vi "Measurement Logic.vi"() -> ()   [LabVIEW 2024, in "Line Regulation_Channel Ganging.lvlib"]
uses:
  Line Regulation_Channel Ganging.lvlib
  <vilib>/Plug-In SDKs/Measurements/Measure Call Context/Measure Call Context.lvclass
  Measurement Configuration.ctl
  Measurement Results.ctl
  <instrlib>/niDCPower/nidcpower.llb/niDCPower Source Mode.ctl
  <instrlib>/niDCPower/nidcpower.llb/niDCPower Wait For Event - Event.ctl
  <instrlib>/niDCPower/nidcpower.llb/niDCPower Output Function.ctl
  shared subVIs/Triggers and Events/NIDCPower_channel_ganging - Configure Digital Edge Source Trigger.vi
  shared subVIs/Triggers and Events/NIDCPower_channel_ganging - Configure Digital Edge Measure Trigger.vi
panel:
  out "measurement results":T1
  in  "measurement configuration":T2={"Source master resource name"="", "Load master resource name"="", "Source slave resource names"=["", ""], "Load slave resource names"=["", ""], "Source system configuration"=enum."Parallel", "Source voltage level range"=64.0, "Source limit symmetry"=enum."Asymmetric", "Source current limit range"=-32.0, "Source current limit low"=-64.0, "Source current limit high"=-64.0, "Source transient response"=1038, "Source sense"=1008, "Source start voltage"=1.0, "Source current sweep points/points per decade"=1, "Source stop voltage"=14.0, "Source voltage gain bandwidth"=2000.0, "Source voltage compensation frequency"=3530.0, "Source voltage pole-zero ratio"=2.0, "Load system configuration"=enum."Parallel", "Load current level"=50.0, "Load current level range"=80.0, "Load limit symmetry"=enum."Symmetric", "Load voltage limit range"=6.0, "Load voltage limit low"=0.0, "Load voltage limit high"=inf, "Load transient response"=1038, "Load sense"=1009, "DUT setup time"=1.0, "Source delay"=0.005, "Aperture time"=0.005, "Load current gain bandwidth"=14000.0, "Load current compensation frequency"=180000.0, "Load current pole-zero ratio"=0.3, "Nominal output voltage"=0.005, "Source sweep type"="Logarithmic", "Mode of operation"=enum."Power on the DUT", "Measurement timeout"=0.0} {"Measurement timeout" format="%.3ps"; "Load sense" items=["Local"=1008, "Remote"=1009]; "Load transient response" items=["Slow"=1041, "Normal"=1038, "Fast"=1039, "Custom"=1042]; "Load voltage limit high" format="%#_6p"; "Load voltage limit low" format="%#_6p"; "Load voltage limit range" format="%#_6p"; "Load current level range" format="%#_6p"; "Source start voltage" format="%#_6p"; "Source sense" items=["Local"=1008, "Remote"=1009]; "Source transient response" items=["Slow"=1041, "Normal"=1038, "Fast"=1039, "Custom"=1042]; "Source current limit low" format="%#_6p"}
  out "measure call context out":refnum<class "Measure Call Context.lvclass">
  in  "measure call context in":refnum<class "Measure Call Context.lvclass">
  out "error out":errorcluster
  in  "error in":errorcluster
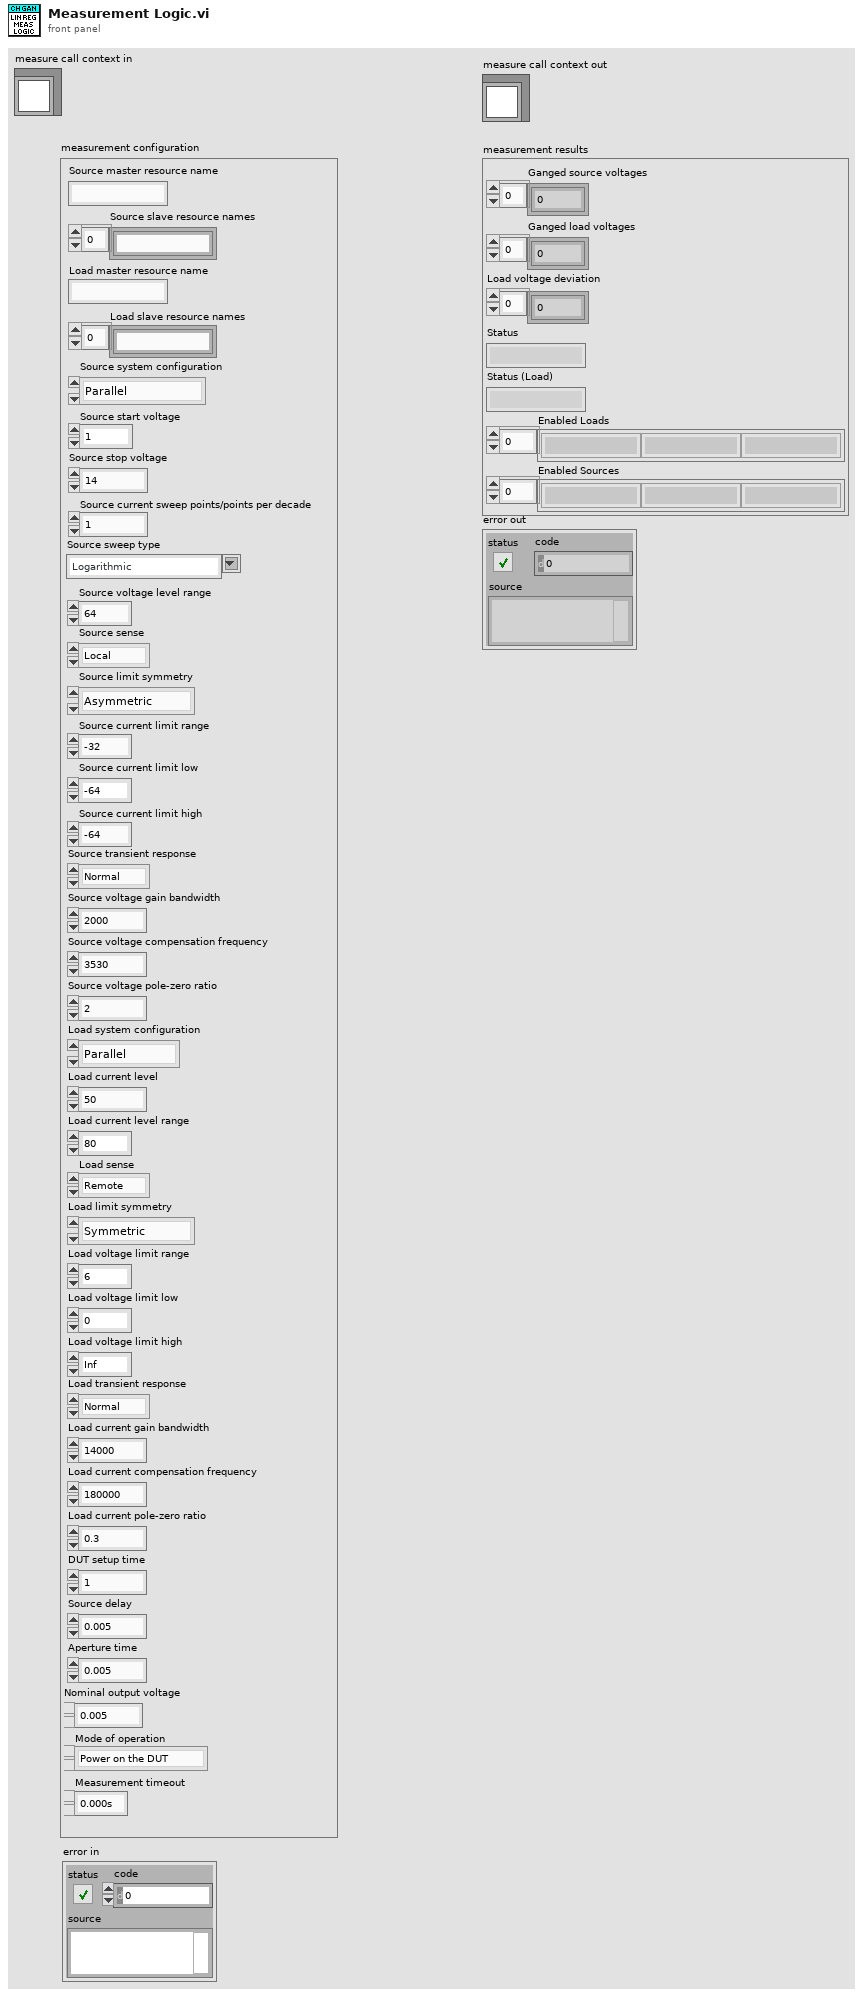
[diagram p1: front panel]
types:
  T1 = typedef "Line Regulation_Channel Ganging.lvlib/Measurement Results.ctl" = cluster{"Ganged source voltages":dbl[], "Ganged load voltages":dbl[], "Load voltage deviation":dbl[], "Status":string, "Status (Load)":string, "Enabled Loads":string[], "Enabled Sources":string[]}
  T2 = typedef "Line Regulation_Channel Ganging.lvlib/Measurement Configuration.ctl" = cluster{"Source master resource name":string, "Load master resource name":string, "Source slave resource names":string[], "Load slave resource names":string[], "Source system configuration":enum32{"Series", "Parallel", "Manual"}, "Source voltage level range":dbl, "Source limit symmetry":enum32{"Symmetric", "Asymmetric"}, "Source current limit range":dbl, "Source current limit low":dbl, "Source current limit high":dbl, "Source transient response":i32, "Source sense":i32, "Source start voltage":dbl, "Source current sweep points/points per decade":i32, "Source stop voltage":dbl, "Source voltage gain bandwidth":dbl, "Source voltage compensation frequency":dbl, "Source voltage pole-zero ratio":dbl, "Load system configuration":enum32{"Series", "Parallel", "Manual"}, "Load current level":dbl, "Load current level range":dbl, "Load limit symmetry":enum32{"Symmetric", "Asymmetric"}, "Load voltage limit range":dbl, "Load voltage limit low":dbl, "Load voltage limit high":dbl, "Load transient response":i32, "Load sense":i32, "DUT setup time":dbl, "Source delay":dbl, "Aperture time":dbl, "Load current gain bandwidth":dbl, "Load current compensation frequency":dbl, "Load current pole-zero ratio":dbl, "Nominal output voltage":dbl, "Source sweep type":string, "Mode of operation":enum32{"Power on the DUT", "Perform measurement", "Power off the DUT"}, "Measurement timeout":dbl}
  T3 = enum32{"Power on the DUT", "Perform measurement", "Power off the DUT"}
  T4 = typedef "niDCPower Output Function.ctl" = i32
  T5 = typedef "niDCPower Source Mode.ctl" = i32
  T6 = typedef "NIDCPower_channel_ganging - ctl - channel def.ctl" = cluster{"resource name":refnum<k15>, "channels":string, "Channel Mode":T7}
  T7 = typedef "NIDCPower_channel_ganging - ctl - channel mode.ctl" = enum32{"Master", "Slave", "Slave - Inverted"}
  T8 = typedef "NIDCPower_channel_ganging - ctl - ganged session.ctl" = cluster{"Ganged Config":T9, "Session List":refnum<k15>[], "Session Mode":T7[], "Channel":string[]}
  T9 = typedef "NIDCPower_channel_ganging - ctl - ganged config.ctl" = enum32{"Series", "Parallel", "Manual"}
  T10 = typedef "niDCPower Wait For Event - Event.ctl" = i32
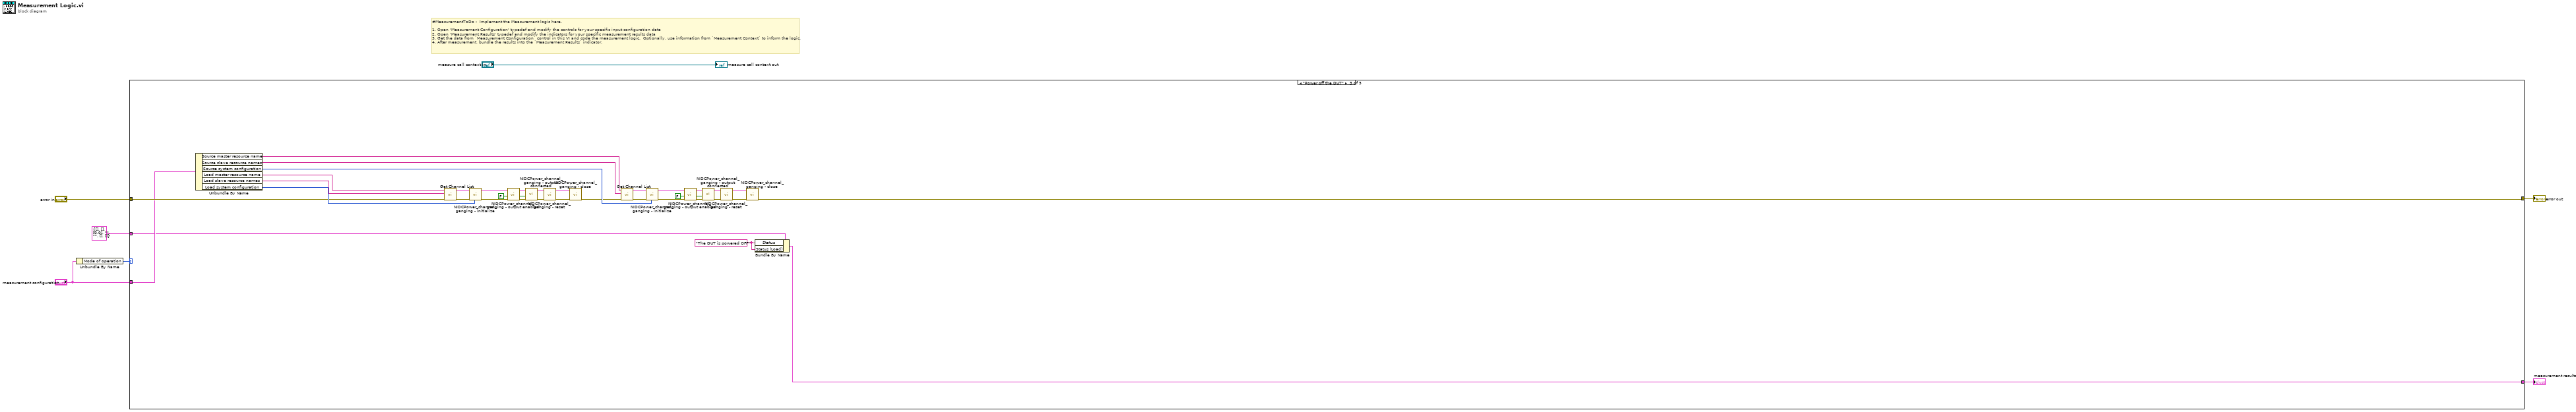
[diagram p0: block diagram]
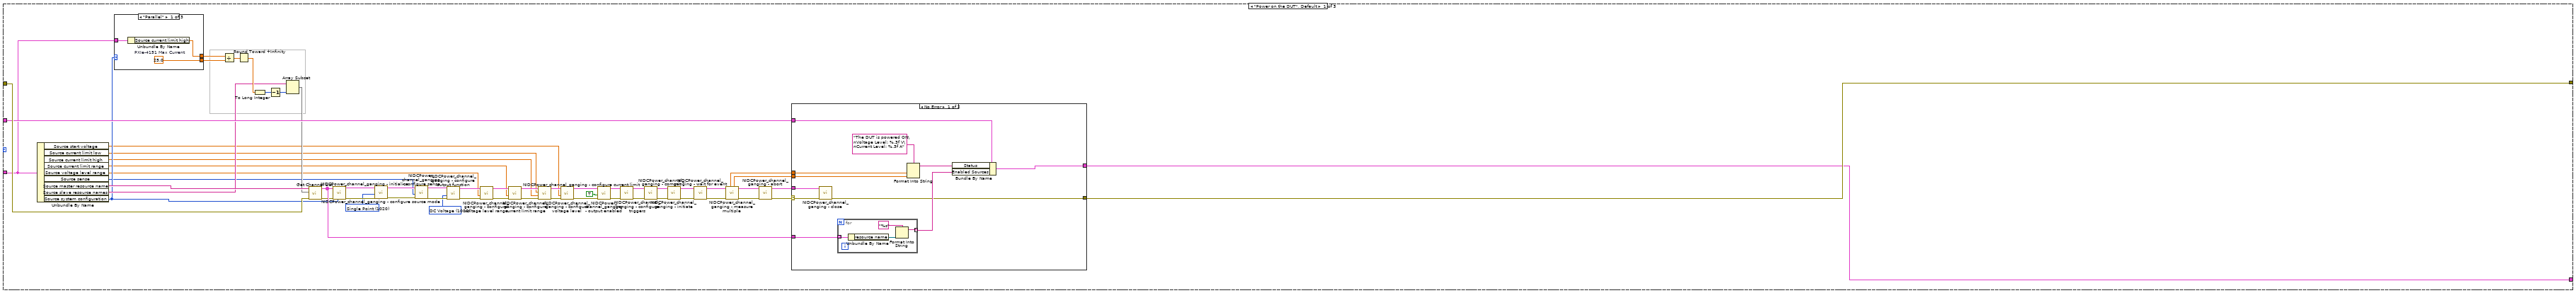
[diagram p2: hidden frame]
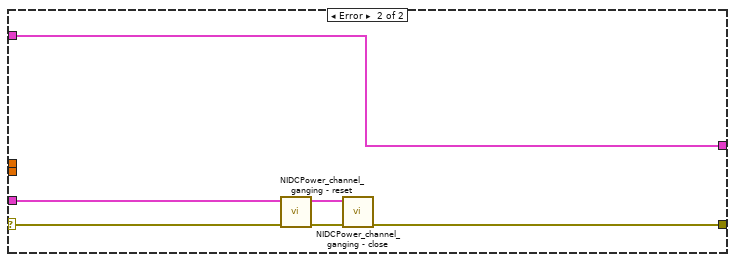
[diagram p3: hidden frame]
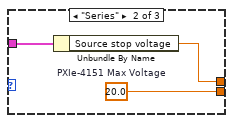
[diagram p4: hidden frame]
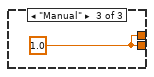
[diagram p5: hidden frame]
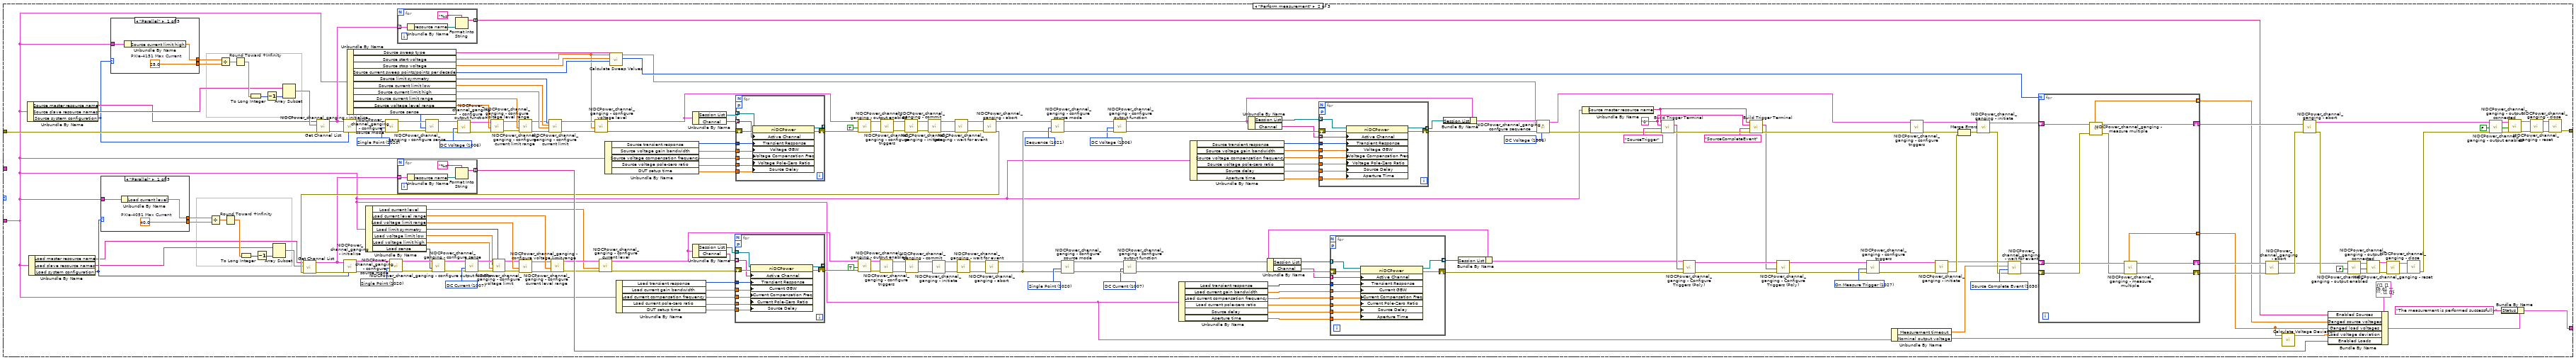
[diagram p6: hidden frame]
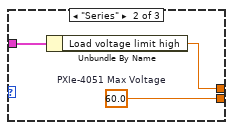
[diagram p7: hidden frame]
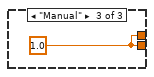
[diagram p8: hidden frame]
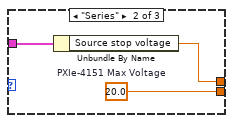
[diagram p9: hidden frame]
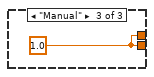
[diagram p10: hidden frame]
diagram:
  # "#MeasurementToDo :  Implement the Measurement logic here.\n\n1. Open 'Measurement Configuration' typedef and modify the controls for your specific input configuration data\n2. Open 'Measurement Results' typedef and modify the indicators for your specific measurement results data\n3. Get the data from `Measurement Configuration` control in this VI and code the measurement logic.  Optionally, use information from `Measurement Context` to inform the logic.\n4. After measurement, bundle the results into the `Measurement Results` indicator."
  n1 = Unbundle By Name("measurement configuration") -> ("Mode of operation"=w3:T3)
  n2 = case shown="\"Power off the DUT\"" w3 {
    tunnel: [w8 w94 w387] -> w6
    tunnel: "measurement configuration" -> [w53 w99 w389]
    tunnel: [w9 w121 w386] -> w5
    tunnel: "error in" -> [w65 w120 w390]
    tunnel: T1 {"Ganged source voltages"=[], "Ganged load voltages"=[], "Load voltage deviation"=[0.0], "Status"="", "Status (Load)"="", "Enabled Loads"=[], "Enabled Sources"=[]} ("Measurement Results") -> [w64 _ w388]
    frame "Power on the DUT", Default {
      w37 = T4 1006 items=["DC Voltage"=1006, "DC Current"=1007, "Pulse Voltage"=1049, "Pulse Current"=1050] ("output function")
      w38 = T5 1020 items=["Single Point"=1020, "Sequence"=1021] ("source mode")
      n3 = Unbundle By Name(w53) -> ("Source start voltage"=w14:dbl, "Source current limit low"=w15:dbl, "Source current limit high"=w17:dbl, "Source current limit range"=w16:dbl, "Source voltage level range"=w19:dbl, "Source sense"=w18:i32, "Source master resource name"=w62:string, "Source slave resource names"=w55:string[], "Source system configuration"=w21:enum32{"Series", "Parallel", "Manual"})
      n4 = case shown="\"Parallel\"" w21 {
        tunnel: [w89 w92 w93] -> w57
        tunnel: w53 -> [w88 w90 _]
        tunnel: [w87 w91 w93] -> w56
        frame "Parallel" {
          w89 = 25.0  # PXIe-4151 Max Current
          n5 = Unbundle By Name(w88) -> ("Source current limit high"=w87:dbl)
        }
        frame "Series" {
          w92 = 20.0  # PXIe-4151 Max Voltage
          n6 = Unbundle By Name(w90) -> ("Source stop voltage"=w91:dbl)
        }
        frame "Manual" {
          w93 = 1.0 ("PXIe-4151 Max Voltage")
        }
      }
      n7 = Divide(x=w56, y=w57) -> (x/y=w59:dbl)
      n8 = Round Toward +Infinity(x=w59) -> (ceil(x): smallest int >= x=w58:dbl)
      n9 = To Long Integer(number=w58) -> (32bit integer=w60:i32)
      n10 = Decrement(x=w60) -> (x-1=w61:i32)
      n11 = Array Subset(array=w55, length=w61) -> (w54:string[])  [unwired: 1 in]
      n12 = call "Get Channel List.vi"("error in (no error)"=w65, "Slave resource names"=w54, "Master resouce name"=w62) -> ("error out"=w20:errorcluster, "Channel List"=w63:T6[])  [unwired: 7 in]
      n13 = call "NIDCPower_channel_ganging - initialize.vi"("Ganged Config"=w21, "error in (no error)"=w20, "Channel List"=w63) -> ("error out"=w51:errorcluster, "Ganged Session Out"=w52:T8)  [unwired: 7 in]
      n14 = call "NIDCPower_channel_ganging - configure source mode.vi"("error in (no error)"=w51, "source mode"=w38, "Ganged Session In"=w52) -> ("error out"=w43:errorcluster, "Ganged Session Out"=w44:T8)  [unwired: 7 in]
      n15 = call "NIDCPower_channel_ganging - configure sense.vi"("error in (no error)"=w43, "sense"=w18, "Ganged Session In"=w44) -> ("error out"=w41:errorcluster, "Ganged Session Out"=w42:T8)  [unwired: 7 in]
      n16 = call "NIDCPower_channel_ganging - configure output function.vi"("error in (no error)"=w41, "output function"=w37, "Ganged Session In"=w42) -> ("error out"=w39:errorcluster, "Ganged Session Out"=w40:T8)  [unwired: 7 in]
      n17 = call "NIDCPower_channel_ganging - configure voltage level range.vi"("error in (no error)"=w39, "voltage level range"=w19, "Ganged Session In"=w40) -> ("error out"=w47:errorcluster, "Ganged Session Out"=w50:T8)  [unwired: 7 in]
      n18 = call "NIDCPower_channel_ganging - configure current limit range.vi"("error in (no error)"=w47, "current limit range"=w16, "Ganged Session In"=w50) -> ("error out"=w46:errorcluster, "Ganged Session Out"=w49:T8)  [unwired: 7 in]
      n19 = call "NIDCPower_channel_ganging - configure current limit.vi"("error in (no error)"=w46, "Current limit/hi"=w17, "Current limit lo"=w15, "Ganged Session In"=w49) -> ("error out"=w45:errorcluster, "Ganged Session Out"=w48:T8)  [unwired: 6 in]
      n20 = call "NIDCPower_channel_ganging - configure voltage level.vi"("error in (no error)"=w45, "voltage level"=w14, "Ganged Session In"=w48) -> ("error out"=w26:errorcluster, "Ganged Session Out"=w27:T8)  [unwired: 7 in]
      n21 = call "NIDCPower_channel_ganging - output enabled.vi"("error in (no error)"=w26, "output enabled"=TRUE, "Ganged Session In"=w27) -> ("error out"=w34:errorcluster, "Ganged Session Out"=w33:T8)  [unwired: 7 in]
      n22 = call "NIDCPower_channel_ganging - configure triggers.vi"("error in (no error)"=w34, "Ganged Session In"=w33) -> ("error out"=w36:errorcluster, "Ganged Session Out"=w35:T8)  [unwired: 8 in]
      n23 = call "NIDCPower_channel_ganging - commit.vi"("error in (no error)"=w36, "Ganged Session In"=w35) -> ("error out"=w31:errorcluster, "Ganged Session Out"=w32:T8)  [unwired: 8 in]
      n24 = call "NIDCPower_channel_ganging - initiate.vi"("error in (no error)"=w31, "Ganged Session In"=w32) -> ("error out"=w29:errorcluster, "Ganged Session Out"=w30:T8)  [unwired: 8 in]
      n25 = call "NIDCPower_channel_ganging - wait for event.vi"("error in (no error)"=w29, "Ganged Session in"=w30) -> ("error out"=w24:errorcluster, "Ganged Session Out"=w25:T8)  [unwired: 8 in]
      n26 = call "NIDCPower_channel_ganging - measure multiple.vi"("error in (no error)"=w24, "Ganged Session In"=w25) -> ("error out"=w22:errorcluster, "Ganged Session Out"=w23:T8, "ganged current measurement"=w11:dbl, "ganged voltage measurement"=w10:dbl)  [unwired: 2 in, 4 out]
      n27 = call "NIDCPower_channel_ganging - abort.vi"("error in (no error)"=w22, "Ganged Session In"=w23) -> ("error out"=w13:errorcluster, "Ganged Session Out"=w12:T8)  [unwired: 8 in]
      n28 = case shown="No Error" w13 {
        selector: w13 -> [w74 w84]
        tunnel: w12 -> [w75 w86]
        tunnel: w10 -> [w73 _]
        tunnel: w11 -> [w72 _]
        tunnel: [w69 w82] -> w9
        tunnel: [w68 w81] -> w8
        tunnel: w63 -> [w67 _]
        tunnel: w64 -> [w66 w81]
        frame No Error {
          n29 = call "NIDCPower_channel_ganging - close.vi"("error in (no error)"=w74, "Ganged Session In"=w75) -> ("error out"=w69:errorcluster)  [unwired: 9 in]
          n30 = for {
            tunnel: w67 -> [w80] mode=indexing
            tunnel: [w77] -> w76 mode=indexing
            n31 = Unbundle By Name(w80) -> ("resource name"=w79:refnum<k15>)
            n32 = Format Into String(format string="%s", w79) -> (resulting string=w77:string)  [unwired: 2 in, 1 out]
          }
          n33 = Format Into String(format string="The DUT is powered ON\nVoltage Level: %.3f V\nCurrent Level: %.3f A", w73, w72) -> (resulting string=w70:string)  [unwired: 2 in, 1 out]
          n34 = Bundle By Name(cluster=w66, "Status"=w70, "Enabled Sources"=w76) -> (w68:T1)
        }
        frame Error {
          n35 = call "NIDCPower_channel_ganging - reset.vi"("error in (no error)"=w84, "Ganged Session In"=w86) -> ("error out"=w83:errorcluster, "Ganged Session Out"=w85:T8)  [unwired: 8 in]
          n36 = call "NIDCPower_channel_ganging - close.vi"("error in (no error)"=w83, "Ganged Session In"=w85) -> ("error out"=w82:errorcluster)  [unwired: 9 in]
        }
      }
    }
    frame "Perform measurement" {
      w154 = T4 1006 items=["DC Voltage"=1006, "DC Current"=1007, "Pulse Voltage"=1049, "Pulse Current"=1050] ("output function")
      w171 = "0" ("Channel Name")
      w206 = 1027 items=["Automatically after Source Complete"=1025, "On Demand"=1026, "On Measure Trigger"=1027] ("Measure When")
      w203 = T4 1006 items=["DC Voltage"=1006, "DC Current"=1007, "Pulse Voltage"=1049, "Pulse Current"=1050] ("output function")
      w208 = T5 1021 items=["Single Point"=1020, "Sequence"=1021] ("source mode")
      w209 = T5 1020 items=["Single Point"=1020, "Sequence"=1021] ("source mode")
      w161 = T4 1007 items=["DC Voltage"=1006, "DC Current"=1007, "Pulse Voltage"=1049, "Pulse Current"=1050] ("output function")
      w256 = T10 1030 items=["Source Complete Event"=1030, "Measure Complete Event"=1031, "Sequence Iteration Complete Event"=1032, "Sequence Engine Done Event"=1033, "Pulse Complete Event"=1051, "Ready For Pulse Trigger Event"=1052] ("event")
      w257 = T4 1007 items=["DC Voltage"=1006, "DC Current"=1007, "Pulse Voltage"=1049, "Pulse Current"=1050] ("output function")
      w270 = T4 1006 items=["DC Voltage"=1006, "DC Current"=1007, "Pulse Voltage"=1049, "Pulse Current"=1050] ("output function")
      w276 = FALSE ("output enabled")
      w275 = FALSE ("output enabled")
      w306 = T5 1020 items=["Single Point"=1020, "Sequence"=1021] ("source mode")
      w307 = T5 1020 items=["Single Point"=1020, "Sequence"=1021] ("source mode")
      n37 = Unbundle By Name(w99) -> ("Source master resource name"=w112:string, "Source slave resource names"=w113:string[], "Source system configuration"=w105:enum32{"Series", "Parallel", "Manual"})
      n38 = Unbundle By Name(w99) -> ("Load master resource name"=w102:string, "Load slave resource names"=w103:string[], "Load system configuration"=w104:enum32{"Series", "Parallel", "Manual"})
      n39 = case shown="\"Parallel\"" w104 {
        tunnel: [w319 w322 w323] -> w110
        tunnel: w99 -> [w318 w321 _]
        tunnel: [w317 w320 w323] -> w111
        frame "Parallel" {
          w319 = 40.0  # PXIe-4051 Max Current
          n40 = Unbundle By Name(w318) -> ("Load current level"=w317:dbl)
        }
        frame "Series" {
          w322 = 60.0  # PXIe-4051 Max Voltage
          n41 = Unbundle By Name(w321) -> ("Load voltage limit high"=w320:dbl)
        }
        frame "Manual" {
          w323 = 1.0 ("PXIe-4051 Max Voltage")
        }
      }
      n42 = case shown="\"Parallel\"" w105 {
        tunnel: [w330 w333 w334] -> w118
        tunnel: w99 -> [w329 w331 _]
        tunnel: [w328 w332 w334] -> w119
        frame "Parallel" {
          w330 = 25.0  # PXIe-4151 Max Current
          n43 = Unbundle By Name(w329) -> ("Source current limit high"=w328:dbl)
        }
        frame "Series" {
          w333 = 20.0  # PXIe-4151 Max Voltage
          n44 = Unbundle By Name(w331) -> ("Source stop voltage"=w332:dbl)
        }
        frame "Manual" {
          w334 = 1.0 ("PXIe-4151 Max Voltage")
        }
      }
      n45 = Divide(x=w111, y=w110) -> (x/y=w107:dbl)
      n46 = Divide(x=w119, y=w118) -> (x/y=w116:dbl)
      n47 = Round Toward +Infinity(x=w107) -> (ceil(x): smallest int >= x=w106:dbl)
      n48 = Round Toward +Infinity(x=w116) -> (ceil(x): smallest int >= x=w117:dbl)
      n49 = To Long Integer(number=w106) -> (32bit integer=w108:i32)
      n50 = To Long Integer(number=w117) -> (32bit integer=w115:i32)
      n51 = Decrement(x=w108) -> (x-1=w109:i32)
      n52 = Decrement(x=w115) -> (x-1=w114:i32)
      n53 = Array Subset(array=w103, length=w109) -> (w101:string[])  [unwired: 1 in]
      n54 = Array Subset(array=w113, length=w114) -> (w310:string[])  [unwired: 1 in]
      n55 = call "Get Channel List.vi"("error in (no error)"=w120, "Slave resource names"=w310, "Master resouce name"=w112) -> ("error out"=w166:errorcluster, "Channel List"=w311:T6[])  [unwired: 7 in]
      n56 = call "NIDCPower_channel_ganging - initialize.vi"("Ganged Config"=w105, "error in (no error)"=w166, "Channel List"=w311) -> ("error out"=w308:errorcluster, "Ganged Session Out"=w309:T8)  [unwired: 7 in]
      n57 = Unbundle By Name(w99) -> ("Source sweep type"=w125:string, "Source start voltage"=w126:dbl, "Source stop voltage"=w130:dbl, "Source current sweep points/points per decade"=w129:i32, "Source limit symmetry"=w291:enum32{"Symmetric", "Asymmetric"}, "Source current limit low"=w292:dbl, "Source current limit high"=w293:dbl, "Source current limit range"=w294:dbl, "Source voltage level range"=w295:dbl, "Source sense"=w169:i32)
      n58 = Unbundle By Name(w99) -> ("Load current level"=w176:dbl, "Load current level range"=w286:dbl, "Load voltage limit range"=w287:dbl, "Load limit symmetry"=w290:enum32{"Symmetric", "Asymmetric"}, "Load voltage limit low"=w289:dbl, "Load voltage limit high"=w288:dbl, "Load sense"=w170:i32)
      n59 = call "NIDCPower_channel_ganging - configure source mode.vi"("error in (no error)"=w308, "source mode"=w307, "Ganged Session In"=w309) -> ("error out"=w253:errorcluster, "Ganged Session Out"=w254:T8)  [unwired: 7 in]
      n60 = for {
        tunnel: w311 -> [w327] mode=indexing
        tunnel: [w324] -> w98 mode=indexing
        n61 = Unbundle By Name(w327) -> ("resource name"=w326:refnum<k15>)
        n62 = Format Into String(format string="%s", w326) -> (resulting string=w324:string)  [unwired: 2 in, 1 out]
      }
      n63 = call "NIDCPower_channel_ganging - configure sense.vi"("error in (no error)"=w253, "sense"=w169, "Ganged Session In"=w254) -> ("error out"=w251:errorcluster, "Ganged Session Out"=w252:T8)  [unwired: 7 in]
      n64 = call "NIDCPower_channel_ganging - configure output function.vi"("error in (no error)"=w251, "output function"=w270, "Ganged Session In"=w252) -> ("error out"=w249:errorcluster, "Ganged Session Out"=w250:T8)  [unwired: 7 in]
      n65 = call "NIDCPower_channel_ganging - configure voltage level range.vi"("error in (no error)"=w249, "voltage level range"=w295, "Ganged Session In"=w250) -> ("error out"=w266:errorcluster, "Ganged Session Out"=w269:T8)  [unwired: 7 in]
      n66 = call "NIDCPower_channel_ganging - configure current limit range.vi"("error in (no error)"=w266, "current limit range"=w294, "Ganged Session In"=w269) -> ("error out"=w265:errorcluster, "Ganged Session Out"=w268:T8)  [unwired: 7 in]
      n67 = call "NIDCPower_channel_ganging - configure current limit.vi"("Limit Symmetry"=w291, "error in (no error)"=w265, "Current limit/hi"=w293, "Current limit lo"=w292, "Ganged Session In"=w268) -> ("error out"=w264:errorcluster, "Ganged Session Out"=w267:T8)  [unwired: 5 in]
      n68 = call "NIDCPower_channel_ganging - configure voltage level.vi"("error in (no error)"=w264, "voltage level"=w126, "Ganged Session In"=w267) -> ("error out"=w224:errorcluster, "Ganged Session Out"=w218:T8)  [unwired: 7 in]
      n69 = Unbundle By Name(w99) -> ("Source transient response"=w148:i32, "Source voltage gain bandwidth"=w144:dbl, "Source voltage compensation frequency"=w143:dbl, "Source voltage pole-zero ratio"=w142:dbl, "DUT setup time"=w145:dbl)
      n70 = call "Calculate Sweep Values.vi"("Sweep type"=w125, "Points"=w129, "Stop level"=w130, "Start level"=w126) -> ("Sweep points"=w128:i32, "Sweep values"=w127:dbl[])  [unwired: 5 in, 1 out]
      n71 = Unbundle By Name(w99) -> ("Load transient response"=w147:i32, "Load current gain bandwidth"=w141:dbl, "Load current compensation frequency"=w140:dbl, "Load current pole-zero ratio"=w139:dbl, "DUT setup time"=w146:dbl)
      n72 = Unbundle By Name(w218) -> ("Session List"=w222:refnum<k15>[], "Channel"=w221:string[])
      n73 = for {
        tunnel: [w374] -> _ mode=indexing
        shift-right: [w372] -> w223
        shift-left: w224 -> [w373]
        workers-P: _ -> [_]
        tunnel: w222 -> [w371] mode=indexing
        tunnel: w221 -> [w370] mode=indexing
        tunnel: w148 -> [w369]
        tunnel: w145 -> [w368]
        tunnel: w144 -> [w367]
        tunnel: w143 -> [w366]
        tunnel: w142 -> [w365]
        n74 = property class="niDCPower"(reference=w371, error in=w373, "Active Channel"=w370, "Transient Response"=w369, "Voltage GBW"=w367, "Voltage Compensation Freq"=w366, "Voltage Pole-Zero Ratio"=w365, "Source Delay"=w368) -> (reference out=w374:refnum<k15>, error out=w372:errorcluster)
      }
      n75 = call "NIDCPower_channel_ganging - output enabled.vi"("error in (no error)"=w223, "output enabled"=TRUE, "Ganged Session In"=w218) -> ("error out"=w227:errorcluster, "Ganged Session Out"=w228:T8)  [unwired: 7 in]
      n76 = call "NIDCPower_channel_ganging - configure triggers.vi"("error in (no error)"=w227, "Ganged Session In"=w228) -> ("error out"=w225:errorcluster, "Ganged Session Out"=w226:T8)  [unwired: 8 in]
      n77 = call "NIDCPower_channel_ganging - commit.vi"("error in (no error)"=w225, "Ganged Session In"=w226) -> ("error out"=w234:errorcluster, "Ganged Session Out"=w233:T8)  [unwired: 8 in]
      n78 = call "NIDCPower_channel_ganging - initiate.vi"("error in (no error)"=w234, "Ganged Session In"=w233) -> ("error out"=w236:errorcluster, "Ganged Session Out"=w235:T8)  [unwired: 8 in]
      n79 = call "NIDCPower_channel_ganging - wait for event.vi"("error in (no error)"=w236, "Ganged Session in"=w235) -> ("error out"=w238:errorcluster, "Ganged Session Out"=w237:T8)  [unwired: 8 in]
      n80 = call "NIDCPower_channel_ganging - abort.vi"("error in (no error)"=w238, "Ganged Session In"=w237) -> ("error out"=w164:errorcluster, "Ganged Session Out"=w207:T8)  [unwired: 8 in]
      n81 = call "Get Channel List.vi"("error in (no error)"=w164, "Slave resource names"=w101, "Master resouce name"=w102) -> ("error out"=w165:errorcluster, "Channel List"=w100:T6[])  [unwired: 7 in]
      n82 = call "NIDCPower_channel_ganging - initialize.vi"("Ganged Config"=w104, "error in (no error)"=w165, "Channel List"=w100) -> ("error out"=w305:errorcluster, "Ganged Session Out"=w304:T8)  [unwired: 7 in]
      n83 = call "NIDCPower_channel_ganging - configure source mode.vi"("error in (no error)"=w305, "source mode"=w306, "Ganged Session In"=w304) -> ("error out"=w247:errorcluster, "Ganged Session Out"=w248:T8)  [unwired: 7 in]
      n84 = for {
        tunnel: w100 -> [w316] mode=indexing
        tunnel: [w313] -> w312 mode=indexing
        n85 = Unbundle By Name(w316) -> ("resource name"=w315:refnum<k15>)
        n86 = Format Into String(format string="%s", w315) -> (resulting string=w313:string)  [unwired: 2 in, 1 out]
      }
      n87 = call "NIDCPower_channel_ganging - configure sense.vi"("error in (no error)"=w247, "sense"=w170, "Ganged Session In"=w248) -> ("error out"=w245:errorcluster, "Ganged Session Out"=w246:T8)  [unwired: 7 in]
      n88 = call "NIDCPower_channel_ganging - configure output function.vi"("error in (no error)"=w245, "output function"=w257, "Ganged Session In"=w246) -> ("error out"=w302:errorcluster, "Ganged Session Out"=w303:T8)  [unwired: 7 in]
      n89 = call "NIDCPower_channel_ganging - configure voltage limit.vi"("Limit Symmetry"=w290, "error in (no error)"=w302, "voltage limit/hi"=w288, "voltage limit lo"=w289, "Ganged Session In"=w303) -> ("error out"=w262:errorcluster, "Ganged Session Out"=w263:T8)  [unwired: 5 in]
      n90 = call "NIDCPower_channel_ganging - configure voltage limit range.vi"("error in (no error)"=w262, "voltage level range"=w287, "Ganged Session In"=w263) -> ("error out"=w260:errorcluster, "Ganged Session Out"=w261:T8)  [unwired: 7 in]
      n91 = call "NIDCPower_channel_ganging - configure current level range.vi"("error in (no error)"=w260, "current level range"=w286, "Ganged Session In"=w261) -> ("error out"=w258:errorcluster, "Ganged Session Out"=w259:T8)  [unwired: 7 in]
      n92 = call "NIDCPower_channel_ganging - configure current level.vi"("error in (no error)"=w258, "current level"=w176, "Ganged Session In"=w259) -> ("error out"=w220:errorcluster, "Ganged Session Out"=w217:T8)  [unwired: 7 in]
      n93 = Unbundle By Name(w217) -> ("Session List"=w216:refnum<k15>[], "Channel"=w215:string[])
      n94 = for {
        tunnel: [w364] -> _ mode=indexing
        shift-right: [w362] -> w219
        shift-left: w220 -> [w363]
        workers-P: _ -> [_]
        tunnel: w216 -> [w361] mode=indexing
        tunnel: w215 -> [w360] mode=indexing
        tunnel: w147 -> [w359]
        tunnel: w146 -> [w358]
        tunnel: w141 -> [w357]
        tunnel: w140 -> [w356]
        tunnel: w139 -> [w355]
        n95 = property class="niDCPower"(reference=w361, error in=w363, "Active Channel"=w360, "Transient Response"=w359, "Current GBW"=w357, "Current Compensation Freq"=w356, "Current Pole-Zero Ratio"=w355, "Source Delay"=w358) -> (reference out=w364:refnum<k15>, error out=w362:errorcluster)
      }
      n96 = call "NIDCPower_channel_ganging - output enabled.vi"("error in (no error)"=w219, "output enabled"=TRUE, "Ganged Session In"=w217) -> ("error out"=w231:errorcluster, "Ganged Session Out"=w232:T8)  [unwired: 7 in]
      n97 = call "NIDCPower_channel_ganging - configure triggers.vi"("error in (no error)"=w231, "Ganged Session In"=w232) -> ("error out"=w229:errorcluster, "Ganged Session Out"=w230:T8)  [unwired: 8 in]
      n98 = call "NIDCPower_channel_ganging - commit.vi"("error in (no error)"=w229, "Ganged Session In"=w230) -> ("error out"=w243:errorcluster, "Ganged Session Out"=w244:T8)  [unwired: 8 in]
      n99 = call "NIDCPower_channel_ganging - initiate.vi"("error in (no error)"=w243, "Ganged Session In"=w244) -> ("error out"=w241:errorcluster, "Ganged Session Out"=w242:T8)  [unwired: 8 in]
      n100 = call "NIDCPower_channel_ganging - wait for event.vi"("error in (no error)"=w241, "Ganged Session in"=w242) -> ("error out"=w239:errorcluster, "Ganged Session Out"=w240:T8)  [unwired: 8 in]
      n101 = call "NIDCPower_channel_ganging - abort.vi"("error in (no error)"=w239, "Ganged Session In"=w240) -> ("error out"=w181:errorcluster, "Ganged Session Out"=w210:T8)  [unwired: 8 in]
      n102 = call "NIDCPower_channel_ganging - configure source mode.vi"("error in (no error)"=w181, "source mode"=w208, "Ganged Session In"=w207) -> ("error out"=w211:errorcluster, "Ganged Session Out"=w212:T8)  [unwired: 7 in]
      n103 = call "NIDCPower_channel_ganging - configure source mode.vi"("error in (no error)"=w181, "source mode"=w209, "Ganged Session In"=w210) -> ("error out"=w214:errorcluster, "Ganged Session Out"=w213:T8)  [unwired: 7 in]
      n104 = call "NIDCPower_channel_ganging - configure output function.vi"("error in (no error)"=w211, "output function"=w203, "Ganged Session In"=w212) -> ("error out"=w204:errorcluster, "Ganged Session Out"=w205:T8)  [unwired: 7 in]
      n105 = call "NIDCPower_channel_ganging - configure output function.vi"("error in (no error)"=w214, "output function"=w161, "Ganged Session In"=w213) -> ("error out"=w186:errorcluster, "Ganged Session Out"=w187:T8)  [unwired: 7 in]
      n106 = Unbundle By Name(w99) -> ("Load transient response"=w153:i32, "Load current gain bandwidth"=w135:dbl, "Load current compensation frequency"=w134:dbl, "Load current pole-zero ratio"=w133:dbl, "Source delay"=w152:dbl, "Aperture time"=w151:dbl)
      n107 = Unbundle By Name(w99) -> ("Source transient response"=w155:i32, "Source voltage gain bandwidth"=w138:dbl, "Source voltage compensation frequency"=w137:dbl, "Source voltage pole-zero ratio"=w136:dbl, "Source delay"=w150:dbl, "Aperture time"=w149:dbl)
      n108 = Unbundle By Name(w205) -> ("Session List"=w299:refnum<k15>[], "Channel"=w185:string[])
      n109 = Unbundle By Name(w187) -> ("Session List"=w184:refnum<k15>[], "Channel"=w183:string[])
      n110 = for {
        tunnel: [w385] -> w298 mode=indexing
        shift-right: [w383] -> w158
        shift-left: w204 -> [w384]
        workers-P: _ -> [_]
        tunnel: w299 -> [w382] mode=indexing
        tunnel: w185 -> [w381] mode=indexing
        tunnel: w155 -> [w380]
        tunnel: w150 -> [w379]
        tunnel: w149 -> [w378]
        tunnel: w138 -> [w377]
        tunnel: w137 -> [w376]
        tunnel: w136 -> [w375]
        n111 = property class="niDCPower"(reference=w382, error in=w384, "Active Channel"=w381, "Transient Response"=w380, "Voltage GBW"=w377, "Voltage Compensation Freq"=w376, "Voltage Pole-Zero Ratio"=w375, "Source Delay"=w379, "Aperture Time"=w378) -> (reference out=w385:refnum<k15>, error out=w383:errorcluster)
      }
      n112 = for {
        tunnel: [w354] -> w182 mode=indexing
        shift-right: [w352] -> w162
        shift-left: w186 -> [w353]
        workers-P: _ -> [_]
        tunnel: w184 -> [w351] mode=indexing
        tunnel: w183 -> [w350] mode=indexing
        tunnel: w153 -> [w349]
        tunnel: w152 -> [w348]
        tunnel: w151 -> [w347]
        tunnel: w135 -> [w346]
        tunnel: w134 -> [w345]
        tunnel: w133 -> [w344]
        n113 = property class="niDCPower"(reference=w351, error in=w353, "Active Channel"=w350, "Transient Response"=w349, "Current GBW"=w346, "Current Compensation Freq"=w345, "Current Pole-Zero Ratio"=w344, "Source Delay"=w348, "Aperture Time"=w347) -> (reference out=w354:refnum<k15>, error out=w352:errorcluster)
      }
      n114 = Bundle By Name(cluster=w205, "Session List"=w298) -> (w160:T8)
      n115 = Bundle By Name(cluster=w187, "Session List"=w182) -> (w163:T8)
      n116 = call "NIDCPower_channel_ganging - confgure sequence.vi"("output function"=w154, "error in (no error)"=w158, "Values"=w127, "Ganged Session In"=w160) -> ("error out"=w157:errorcluster, "Ganged Session Out"=w159:T8)  [unwired: 6 in]
      n117 = Unbundle By Name(w99) -> ("Source master resource name"=w156:string)
      n118 = call "Build Trigger Terminal.vi"("error in (no error)"=w157, "Trigger/Event Name"="SourceTrigger", "Channel Name"=w171, "Resource Name"=w156) -> ("error out"=w180:errorcluster, "Terminal Name"=w168:string)  [unwired: 6 in]
      n119 = call-poly "NIDCPower_channel_ganging - Configure Triggers (Poly).vi"("error in (no error)"=w162, "output terminal"=w168, "Ganged Session in"=w163) -> ("error out"=w172:errorcluster, "Ganged Session out"=w173:T8)  [unwired: 7 in]
      n120 = call "Build Trigger Terminal.vi"("error in (no error)"=w180, "Trigger/Event Name"="SourceCompleteEvent", "Channel Name"=w171, "Resource Name"=w156) -> ("error out"=w179:errorcluster, "Terminal Name"=w167:string)  [unwired: 6 in]
      n121 = call-poly "NIDCPower_channel_ganging - Configure Triggers (Poly).vi"("error in (no error)"=w172, "output terminal"=w167, "Ganged Session in"=w173) -> ("error out"=w174:errorcluster, "Ganged Session out"=w175:T8)  [unwired: 7 in]
      n122 = call "NIDCPower_channel_ganging - configure triggers.vi"("error in (no error)"=w174, "Measure When"=w206, "Ganged Session In"=w175) -> ("error out"=w296:errorcluster, "Ganged Session Out"=w297:T8)  [unwired: 7 in]
      n123 = Unbundle By Name(w99) -> ("Measurement timeout"=w97:dbl, "Nominal output voltage"=w124:dbl)
      n124 = call "NIDCPower_channel_ganging - configure triggers.vi"("error in (no error)"=w179, "Ganged Session In"=w159) -> ("error out"=w272:errorcluster, "Ganged Session Out"=w273:T8)  [unwired: 8 in]
      n125 = call "NIDCPower_channel_ganging - initiate.vi"("error in (no error)"=w296, "Ganged Session In"=w297) -> ("error out"=w271:errorcluster, "Ganged Session Out"=w255:T8)  [unwired: 8 in]
      n126 = Merge Errors(w272, w271) -> (w274:errorcluster)
      n127 = call "NIDCPower_channel_ganging - initiate.vi"("error in (no error)"=w274, "Ganged Session In"=w273) -> ("error out"=w202:errorcluster, "Ganged Session Out"=w189:T8)  [unwired: 8 in]
      n128 = call "NIDCPower_channel_ganging - wait for event.vi"("error in (no error)"=w202, "event"=w256, "timeout (10.0)"=w97, "Ganged Session in"=w255) -> ("error out"=w193:errorcluster, "Ganged Session Out"=w191:T8)  [unwired: 6 in]
      n129 = for {
        N: w128 -> [_]
        shift-right: [w342] -> w192
        shift-left: w193 -> [w343]
        shift-right: [w340] -> w190
        shift-left: w191 -> [w341]
        shift-right: [w338] -> w188
        shift-left: w189 -> [w339]
        tunnel: [w336] -> w131 mode=indexing
        tunnel: [w335] -> w123 mode=indexing
        n130 = call "NIDCPower_channel_ganging - measure multiple.vi"("error in (no error)"=w343, "Ganged Session In"=w339) -> ("error out"=w337:errorcluster, "Ganged Session Out"=w338:T8, "ganged voltage measurement"=w336:dbl)  [unwired: 2 in, 5 out]
        n131 = call "NIDCPower_channel_ganging - measure multiple.vi"("error in (no error)"=w337, "Ganged Session In"=w341) -> ("error out"=w342:errorcluster, "Ganged Session Out"=w340:T8, "ganged voltage measurement"=w335:dbl)  [unwired: 2 in, 5 out]
      }
      n132 = call "NIDCPower_channel_ganging - abort.vi"("error in (no error)"=w192, "Ganged Session In"=w190) -> ("error out"=w285:errorcluster, "Ganged Session Out"=w281:T8)  [unwired: 8 in]
      n133 = call "Calculate Voltage Deviation.vi"("Nominal output voltage"=w124, "Voltage measurements"=w123) -> ("Load voltage deviation"=w122:dbl[])  [unwired: 9 in]
      n134 = call "NIDCPower_channel_ganging - abort.vi"("error in (no error)"=w285, "Ganged Session In"=w188) -> ("error out"=w284:errorcluster, "Ganged Session Out"=w277:T8)  [unwired: 8 in]
      n135 = Bundle By Name(cluster=T1 {"Ganged source voltages"=[], "Ganged load voltages"=[], "Load voltage deviation"=[0.0], "Status"="", "Status (Load)"="", "Enabled Loads"=[], "Enabled Sources"=[]} ("Measurement Results"), "Enabled Sources"=w98, "Ganged source voltages"=w131, "Ganged load voltages"=w123, "Load voltage deviation"=w122, "Enabled Loads"=w312) -> (w96:T1)
      n136 = call "NIDCPower_channel_ganging - output enabled.vi"("error in (no error)"=w284, "output enabled"=w276, "Ganged Session In"=w281) -> ("error out"=w282:errorcluster, "Ganged Session Out"=w283:T8)  [unwired: 7 in]
      n137 = call "NIDCPower_channel_ganging - output connected.vi"("error in (no error)"=w282, "output enabled"=w276, "Ganged Session In"=w283) -> ("error out"=w201:errorcluster, "Ganged Session Out"=w200:T8)  [unwired: 7 in]
      n138 = call "NIDCPower_channel_ganging - reset.vi"("error in (no error)"=w201, "Ganged Session In"=w200) -> ("error out"=w198:errorcluster, "Ganged Session Out"=w199:T8)  [unwired: 8 in]
      n139 = call "NIDCPower_channel_ganging - close.vi"("error in (no error)"=w198, "Ganged Session In"=w199) -> ("error out"=w278:errorcluster)  [unwired: 9 in]
      n140 = call "NIDCPower_channel_ganging - output enabled.vi"("error in (no error)"=w278, "output enabled"=w275, "Ganged Session In"=w277) -> ("error out"=w280:errorcluster, "Ganged Session Out"=w279:T8)  [unwired: 7 in]
      n141 = Bundle By Name(cluster=w96, "Status"="The measurement is performed successfully") -> (w94:T1)
      n142 = call "NIDCPower_channel_ganging - output connected.vi"("error in (no error)"=w280, "output enabled"=w275, "Ganged Session In"=w279) -> ("error out"=w196:errorcluster, "Ganged Session Out"=w197:T8)  [unwired: 7 in]
      n143 = call "NIDCPower_channel_ganging - reset.vi"("error in (no error)"=w196, "Ganged Session In"=w197) -> ("error out"=w194:errorcluster, "Ganged Session Out"=w195:T8)  [unwired: 8 in]
      n144 = call "NIDCPower_channel_ganging - close.vi"("error in (no error)"=w194, "Ganged Session In"=w195) -> ("error out"=w121:errorcluster)  [unwired: 9 in]
    }
    frame "Power off the DUT" {
      w391 = "The DUT is powered OFF"
      w399 = FALSE ("output enabled")
      w415 = FALSE ("output enabled")
      n145 = Unbundle By Name(w389) -> ("Source master resource name"=w393:string, "Source slave resource names"=w392:string[], "Source system configuration"=w420:enum32{"Series", "Parallel", "Manual"}, "Load master resource name"=w414:string, "Load slave resource names"=w413:string[], "Load system configuration"=w410:enum32{"Series", "Parallel", "Manual"})
      n146 = call "Get Channel List.vi"("error in (no error)"=w390, "Slave resource names"=w413, "Master resouce name"=w414) -> ("error out"=w411:errorcluster, "Channel List"=w412:T6[])  [unwired: 7 in]
      n147 = call "NIDCPower_channel_ganging - initialize.vi"("Ganged Config"=w410, "error in (no error)"=w411, "Channel List"=w412) -> ("error out"=w409:errorcluster, "Ganged Session Out"=w408:T8)  [unwired: 7 in]
      n148 = call "NIDCPower_channel_ganging - output enabled.vi"("error in (no error)"=w409, "output enabled"=w415, "Ganged Session In"=w408) -> ("error out"=w417:errorcluster, "Ganged Session Out"=w416:T8)  [unwired: 7 in]
      n149 = call "NIDCPower_channel_ganging - output connected.vi"("error in (no error)"=w417, "output enabled"=w415, "Ganged Session In"=w416) -> ("error out"=w418:errorcluster, "Ganged Session Out"=w419:T8)  [unwired: 7 in]
      n150 = call "NIDCPower_channel_ganging - reset.vi"("error in (no error)"=w418, "Ganged Session In"=w419) -> ("error out"=w406:errorcluster, "Ganged Session Out"=w407:T8)  [unwired: 8 in]
      n151 = call "NIDCPower_channel_ganging - close.vi"("error in (no error)"=w406, "Ganged Session In"=w407) -> ("error out"=w394:errorcluster)  [unwired: 9 in]
      n152 = call "Get Channel List.vi"("error in (no error)"=w394, "Slave resource names"=w392, "Master resouce name"=w393) -> ("error out"=w401:errorcluster, "Channel List"=w400:T6[])  [unwired: 7 in]
      n153 = call "NIDCPower_channel_ganging - initialize.vi"("Ganged Config"=w420, "error in (no error)"=w401, "Channel List"=w400) -> ("error out"=w402:errorcluster, "Ganged Session Out"=w403:T8)  [unwired: 7 in]
      n154 = call "NIDCPower_channel_ganging - output enabled.vi"("error in (no error)"=w402, "output enabled"=w399, "Ganged Session In"=w403) -> ("error out"=w397:errorcluster, "Ganged Session Out"=w398:T8)  [unwired: 7 in]
      n155 = call "NIDCPower_channel_ganging - output connected.vi"("error in (no error)"=w397, "output enabled"=w399, "Ganged Session In"=w398) -> ("error out"=w396:errorcluster, "Ganged Session Out"=w395:T8)  [unwired: 7 in]
      n156 = call "NIDCPower_channel_ganging - reset.vi"("error in (no error)"=w396, "Ganged Session In"=w395) -> ("error out"=w405:errorcluster, "Ganged Session Out"=w404:T8)  [unwired: 8 in]
      n157 = call "NIDCPower_channel_ganging - close.vi"("error in (no error)"=w405, "Ganged Session In"=w404) -> ("error out"=w386:errorcluster)  [unwired: 9 in]
      n158 = Bundle By Name(cluster=w388, "Status"=w391, "Status (Load)"=w391) -> (w387:T1)
    }
  }
  "error out" <- w5
  "measurement results" <- w6
  "measure call context out" <- "measure call context in"
